vi "Windspeed Warnings.vi"() -> ()   [LabVIEW 2022 SP3]
uses:
  Control 1.ctl
panel:
  out "Weather Data Out":T1={"Current Temperature"=0.0, "Max Temperature"=0.0, "Min Temperature"=0.0, "Warning?"=FALSE, "Warning Text"="No Warning", "Current Windspeed"=0.0, "Max Windspeed"=0.0, "Windspeed Warning?"=FALSE, "Windspeed Warning Text"="No Warning"}
  in  "Weather Data In":T1={"Current Temperature"=0.0, "Max Temperature"=0.0, "Min Temperature"=0.0, "Warning?"=FALSE, "Warning Text"="No Warning", "Current Windspeed"=0.0, "Max Windspeed"=0.0, "Windspeed Warning?"=FALSE, "Windspeed Warning Text"="No Warning"}
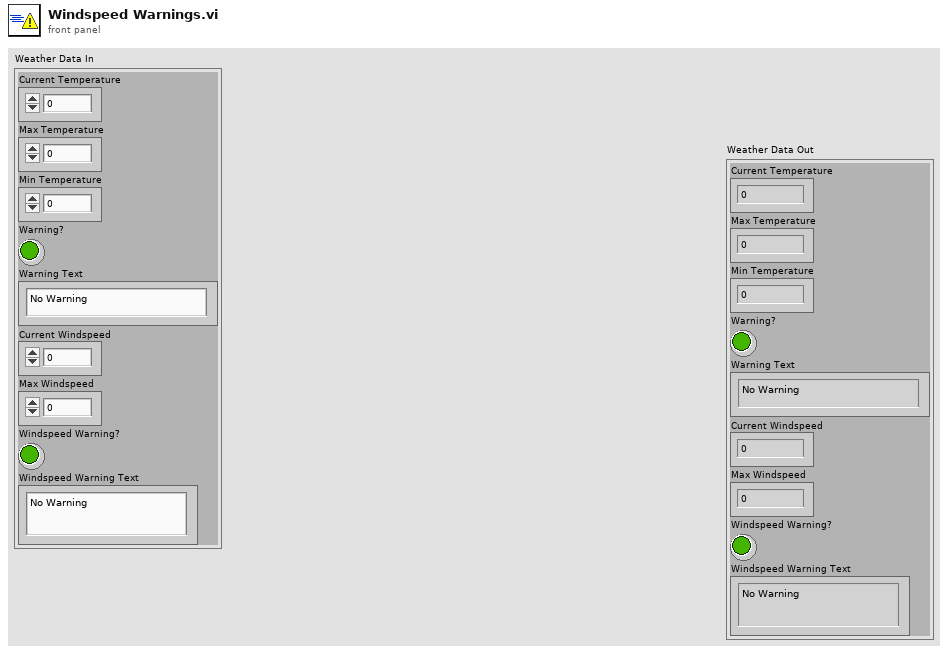
[diagram p1: front panel]
types:
  T1 = typedef "Control 1.ctl" = cluster{"Current Temperature":dbl, "Max Temperature":dbl, "Min Temperature":dbl, "Warning?":bool, "Warning Text":string, "Current Windspeed":dbl, "Max Windspeed":dbl, "Windspeed Warning?":bool, "Windspeed Warning Text":string}
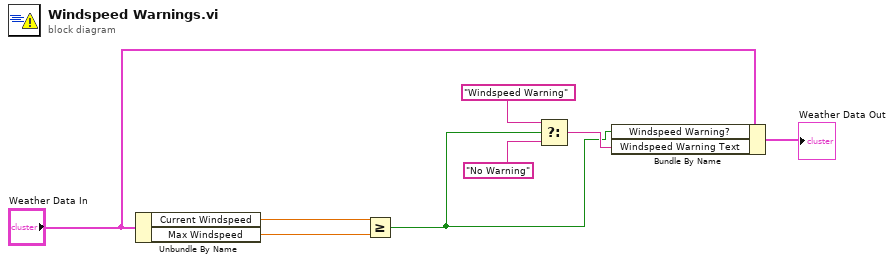
[diagram p0: block diagram]
diagram:
  n1 = Unbundle By Name("Weather Data In") -> ("Current Windspeed"=w6:dbl, "Max Windspeed"=w5:dbl)
  n2 = Greater Or Equal?(x=w6, y=w5) -> (x >= y?=w1:bool)
  n3 = Select(t="Windspeed Warning", s=w1, f="No Warning") -> (s? t:f=w2:string)
  n4 = Bundle By Name(cluster="Weather Data In", "Windspeed Warning?"=w1, "Windspeed Warning Text"=w2) -> (→"Weather Data Out":T1)
